vi "WristDirectionSelection.vi"(10 "Wrist Back":bool, 11 "Wrist Front":bool) -> ()   [LabVIEW 2018]
uses:
  Robot Global Data.vi
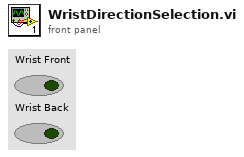
[diagram p1: front panel]
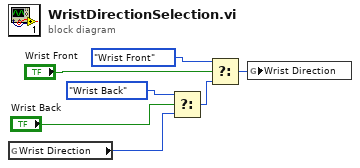
[diagram p0: block diagram]
diagram:
  n1 = global read "Robot Global Data.vi" "Wrist Direction"() -> (w2:enum16{"Wrist Front", "Wrist Back"})
  n2 = Select(t=enum16{"Wrist Front", "Wrist Back"}."Wrist Back" ("Wrist Direction"), s="Wrist Back", f=w2) -> (s? t:f=w6:enum16{"Wrist Front", "Wrist Back"})
  n3 = Select(t=enum16{"Wrist Front", "Wrist Back"}."Wrist Front" ("Wrist Direction"), s="Wrist Front", f=w6) -> (s? t:f=w1:enum16{"Wrist Front", "Wrist Back"})
  n4 = global write "Robot Global Data.vi" "Wrist Direction"(w1) -> ()
